vi "test Import Same Module Same Configuration.vi"(8 "error in (no error)":errorcluster, 11 "TestCase in":refnum<class "SLSC Switch Import Export Unit Tests.lvclass">) -> (0 "error out":errorcluster, 3 "TestCase out":refnum<class "SLSC Switch Import Export Unit Tests.lvclass">)   [LabVIEW 2017, in "SLSC Switch Import Export Unit Tests.lvclass"]
uses:
  SLSC Switch Import Export Unit Tests.lvclass
  <vilib>/addons/_JKI Toolkits/VI Tester/TestCase.llb/TestCase.lvclass
  <vilib>/NI/NI VeriStand Custom Device Import and Export Tool/ImportExport.lvlib
  Scripting/NI-SWITCH Scripting.lvlib
  Shared/VeriStand System Definition Test Utilities/VeriStand System Definition Test Utilities.lvlib
  Shared/Endpoint Configuration Enum.ctl
  Shared/NI-SWITCH Shared.lvlib
  Shared/Endpoint Configuration Cluster.ctl
  C:/Program Files (x86)/National Instruments/LabVIEW 2017/vi.lib/addons/_JKI Toolkits/VI Tester/TestCase.llb/TestCase.lvclass
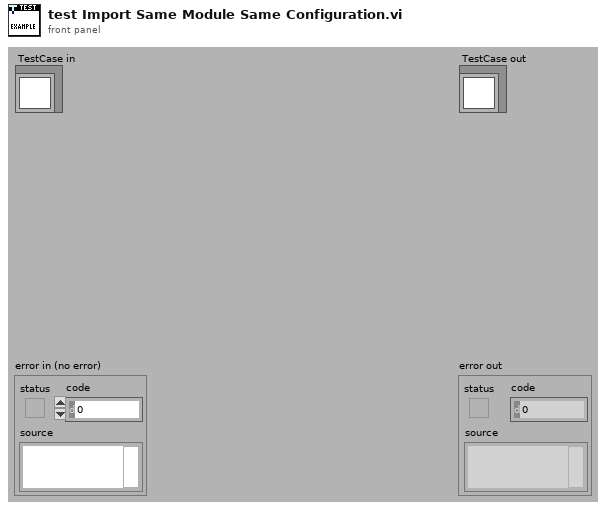
[diagram p1: front panel]
types:
  T1 = cluster{"Ignore Properties":string[], "Ignore Top Level Name":bool}
  T2 = typedef "NI-SWITCH Shared.lvlib/Endpoint Configuration Cluster.ctl" = cluster{"Endpoint":string, "Configuration":T3}
  T3 = typedef "NI-SWITCH Shared.lvlib/Endpoint Configuration Enum.ctl" = enum16{"Load", "Source", "Configuration"}
  T4 = typedef "Custom Device API.lvlib/Custom Device Item Ref.ctl" = u64
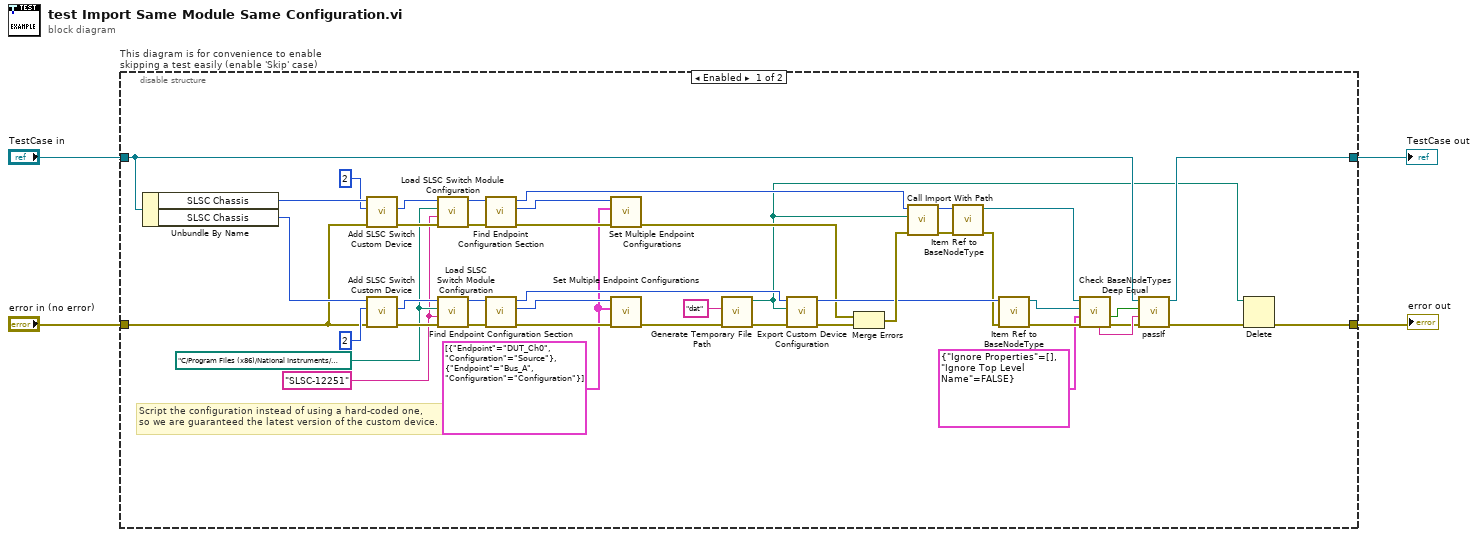
[diagram p0: block diagram]
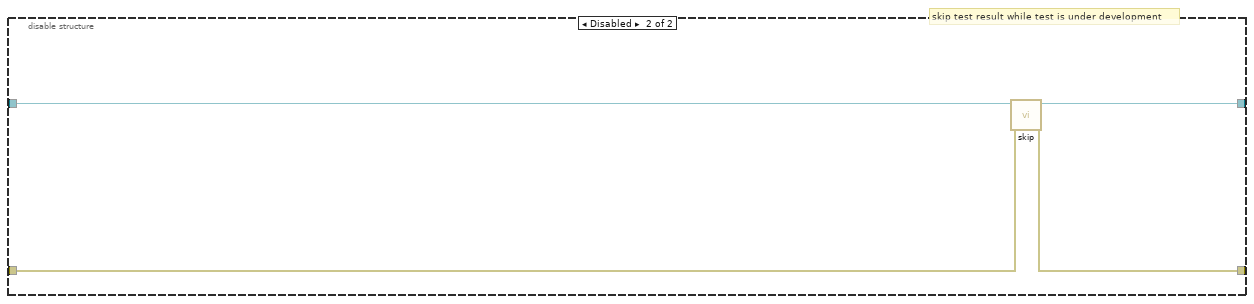
[diagram p2: hidden frame]
diagram:
  n1 = disable-structure "This diagram is for convenience to enable skipping a test easily (enable 'Skip' case)" shown="Enabled" {
    disable-tunnel: "TestCase in" -> [w36 w52]
    disable-tunnel: [w8 w50] -> w1
    disable-tunnel: [w6 w51] -> w3
    disable-tunnel: "error in (no error)" -> [w30 w49]
    frame Enabled {
      w12 = T2[] [{"Endpoint"="DUT_Ch0", "Configuration"=enum."Source"}, {"Endpoint"="Bus_A", "Configuration"=enum."Configuration"}] ("endpoint configurations")
      w16 = path "C:/Program Files (x86)/National Instruments/Shared/NI-SLSC Switch/Modules/SLSC-12251-switches.json" ("switches json file")
      w15 = "SLSC-12251" ("product name")
      # "Script the configuration instead of using a hard-coded one,\nso we are guaranteed the latest version of the custom device."
      n2 = Unbundle By Name(w36) -> ("SLSC Chassis"=w31:u64, "SLSC Chassis"=w48:u64)
      n3 = call "Add SLSC Switch Custom Device.vi"("error in"=w30, "slot number"=u32 2, "slsc chassis in"=w31) -> ("error out"=w18:errorcluster, "slsc switch custom device"=w14:T4)  [unwired: 6 in, 1 out]
      n4 = call "Add SLSC Switch Custom Device.vi"("error in"=w30, "slot number"=u32 2, "slsc chassis in"=w48) -> ("error out"=w29:errorcluster, "slsc switch custom device"=w27:T4)  [unwired: 6 in, 1 out]
      n5 = call "Load SLSC Switch Module Configuration.vi"("error in"=w18, "product name"=w15, "switches json file"=w16, "slsc switch custom device in"=w14) -> ("error out"=w17:errorcluster, "slsc switch custom device out"=w19:T4)  [unwired: 6 in]
      n6 = call "Load SLSC Switch Module Configuration.vi"("error in"=w29, "product name"=w15, "switches json file"=w16, "slsc switch custom device in"=w27) -> ("error out"=w28:errorcluster, "slsc switch custom device out"=w25:T4)  [unwired: 6 in]
      n7 = call "Find Endpoint Configuration Section.vi"("error in"=w17, "slsc switch custom device in"=w19) -> ("error out"=w13:errorcluster, "endpoint configuration"=w11:T4, "slsc switch custom device out"=w10:T4)  [unwired: 7 in]
      n8 = call "Find Endpoint Configuration Section.vi"("error in"=w28, "slsc switch custom device in"=w25) -> ("error out"=w26:errorcluster, "endpoint configuration"=w23:T4, "slsc switch custom device out"=w22:T4)  [unwired: 7 in]
      n9 = call "Set Multiple Endpoint Configurations.vi"("error in"=w13, "endpoint configurations"=w12, "endpoint configuration in"=w11) -> ("error out"=w9:errorcluster)  [unwired: 7 in, 1 out]
      n10 = call "Set Multiple Endpoint Configurations.vi"("error in"=w26, "endpoint configurations"=w12, "endpoint configuration in"=w23) -> ("error out"=w24:errorcluster)  [unwired: 7 in, 1 out]
      n11 = call <vilib>:"Generate Temporary File Path.vi"("error in (no error)"=w24, "Temporary File Extension (tmp)"="dat") -> ("error out"=w45:errorcluster, "Unique Temporary File Path"=w5:path)  [unwired: 8 in]
      n12 = call <vilib>:"Export Custom Device Configuration.vi"("error in (no error)"=w45, "Path"=w5, "ID"=w22) -> ("error out"=w44:errorcluster, "ID out"=w41:u64)  [unwired: 7 in]
      n13 = Merge Errors(w9, w44) -> (w43:errorcluster)
      n14 = call "Call Import With Path.vi"("error in (no error)"=w43, "Path"=w5, "Node Ptr"=w10) -> ("error out"=w40:errorcluster, "Node Ptr out"=w42:u64)  [unwired: 7 in]
      n15 = call "Item Ref to BaseNodeType.vi"("error in (no error)"=w40, "Item Ref"=w42) -> ("error out"=w39:errorcluster, "BaseNodeType"=w33:refnum<k24>)  [unwired: 8 in]
      n16 = call "Item Ref to BaseNodeType.vi"("error in (no error)"=w39, "Item Ref"=w41) -> ("error out"=w38:errorcluster, "BaseNodeType"=w37:refnum<k24>)  [unwired: 8 in]
      n17 = call "Check BaseNodeTypes Deep Equal.vi"("error in (no error)"=w38, "Settings"=T1 {"Ignore Properties"=[], "Ignore Top Level Name"=FALSE}, "BaseNodeType 2"=w37, "BaseNodeType 1"=w33) -> ("error out"=w32:errorcluster, "Equal?"=w35:bool, "Inequality context"=w34:string)  [unwired: 3 in, 2 out]
      n18 = call-dynamic "passIf.vi"("error in (no error)"=w32, "message (\"\")"=w34, "pass"=w35, "TestCase in"=w36) -> ("error out"=w7:errorcluster, "TestCase out"=w8:refnum<class "SLSC Switch Import Export Unit Tests.lvclass">)  [unwired: 6 in]
      n19 = Delete(path (use dialog)=w5, error in=w7) -> (error out=w6:errorcluster)  [unwired: 3 in, 2 out]
    }
    frame Disabled {
      # "skip test result while test is under development"
      n20 = call <vilib>:"skip.vi"("error in (no error)"=w49, "TestCase in"=w52) -> ("error out"=w51:errorcluster, "TestCase out"=w50:refnum<class "SLSC Switch Import Export Unit Tests.lvclass">)  [unwired: 8 in]
    }
  }
  "error out" <- w3
  "TestCase out" <- w1
